vi "Resolve Value Source.vi"(8 "error in (no error)":errorcluster, 10 "Config Element":refnum<class "Config Element.lvclass">, 11 "VolatusAPI in":refnum<class "VolatusAPI.lvclass">) -> (0 "error out":errorcluster, 2 "Source":T1, 3 "VolatusAPI":refnum<class "VolatusAPI.lvclass">, 5 "Constant":dbl, 7 "Channel":refnum<class "Channel DBL.lvclass">)   [LabVIEW 2020, in "VolatusGUIElements.lvlib" / "GaugeIndicator.lvclass"]
uses:
  GaugeIndicator.lvclass
  Volatus/VolatusAPI/VolatusAPI.lvclass
  lv-cdm/CDM-Config/Config Element/Config Element.lvclass
  lv-vecto/Vecto/Channel DBL/Channel DBL.lvclass
  Value Source.ctl
  lv-vecto/Vecto/Group DBL/Group DBL.lvclass
  C:/dev/lv20CE/relink/lv-vecto/Vecto/Group/Group.lvclass
  GaugeIndicator.lvclass/GaugeIndicator.ctl
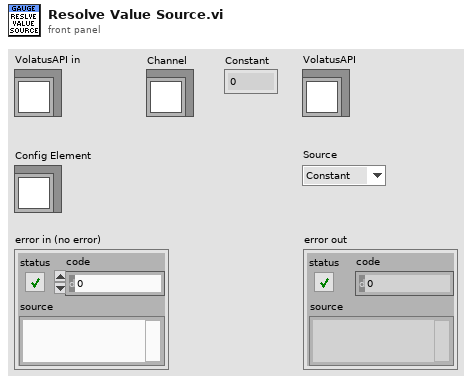
[diagram p1: front panel]
types:
  T1 = typedef "VolatusGUIElements.lvlib/GaugeIndicator.lvclass/Value Source.ctl" = enum16{"Constant", "Channel"}
  T2 = typedef "CDM-Config.lvlib/Value Type.ctl" = enum16{"String", "Number", "Bool", "Object", "Array"}
  T3 = typedef "VectoConfig.lvlib/Channel Info.ctl" = cluster{"Name":string, "Group":string, "Owning Node":string, "Owning Task":string, "Resource":string}
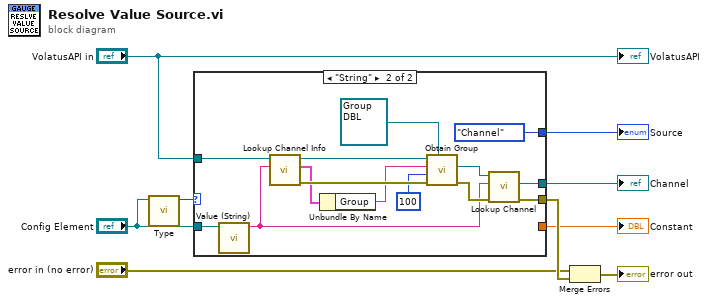
[diagram p0: block diagram]
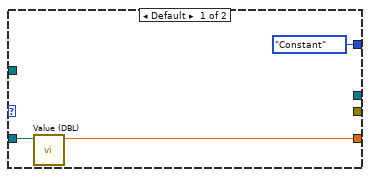
[diagram p2: hidden frame]
diagram:
  n1 = call "Type.vi"("Config Element in"="Config Element") -> ("Value Type"=w8:T2)  [unwired: 9 in, 1 out]
  n2 = case shown="\"String\"" w8 {
    tunnel: "VolatusAPI in" -> [_ w24]
    tunnel: "Config Element" -> [w12 w25]
    tunnel: [_ w16] -> w6
    tunnel: [Value_Source."Constant" ("Source") Value_Source."Channel" ("Source")] -> w5
    tunnel: [_ w14] -> w9
    tunnel: [w11 _] -> w4
    frame Default {
      n3 = call "Value (DBL).vi"("Config Element in"=w12) -> ("DBL Value"=w11:dbl)  [unwired: 9 in, 1 out]
    }
    frame "String" {
      n4 = call "Value (String).vi"("Config Element in"=w25) -> ("String Value"=w17:string)  [unwired: 9 in, 1 out]
      n5 = call "Lookup Channel Info.vi"("Channel Name"=w17, "VolatusAPI in"=w24) -> ("error out"=w26:errorcluster, "Channel Info"=w23:T3, "VolatusAPI out"=w22:refnum<class "VolatusAPI.lvclass">)  [unwired: 6 in, 1 out]
      n6 = Unbundle By Name(w23) -> ("Group"=w20:string)
      n7 = call "Obtain Group.vi"("Group Type (Abstract)"=refnum<class "Group DBL.lvclass"> refnum ("Vecto.lvlib:Group.lvclass"), "error in (no error)"=w26, "Timeout ms (5000)"=u32 100, "Group Name"=w20, "VolatusAPI in"=w22) -> ("error out"=w18:errorcluster, "Group"=w19:refnum<class "Group DBL.lvclass">)  [unwired: 4 in, 1 out]
      n8 = call "Lookup Channel.vi"("error in (no error)"=w18, "Channel Name"=w17, "Group in"=w19) -> ("error out"=w14:errorcluster, "Channel"=w16:refnum<class "Channel DBL.lvclass">)  [unwired: 6 in, 1 out]
    }
  }
  "Channel" <- w6
  "Constant" <- w4
  "Source" <- w5
  n9 = Merge Errors("error in (no error)", w9) -> (→"error out":errorcluster)
  "VolatusAPI" <- "VolatusAPI in"
